vi "Exercise 4.3.vi"() -> ()   [LabVIEW 2010]
panel:
  in  "stop":bool
  in  "Left/Right":i32=-22
  in  "Up/Down":i32=-142
  in  "Scale 2":u32=29 min=1
  out "Intensity Graph":dbl[][](graph)
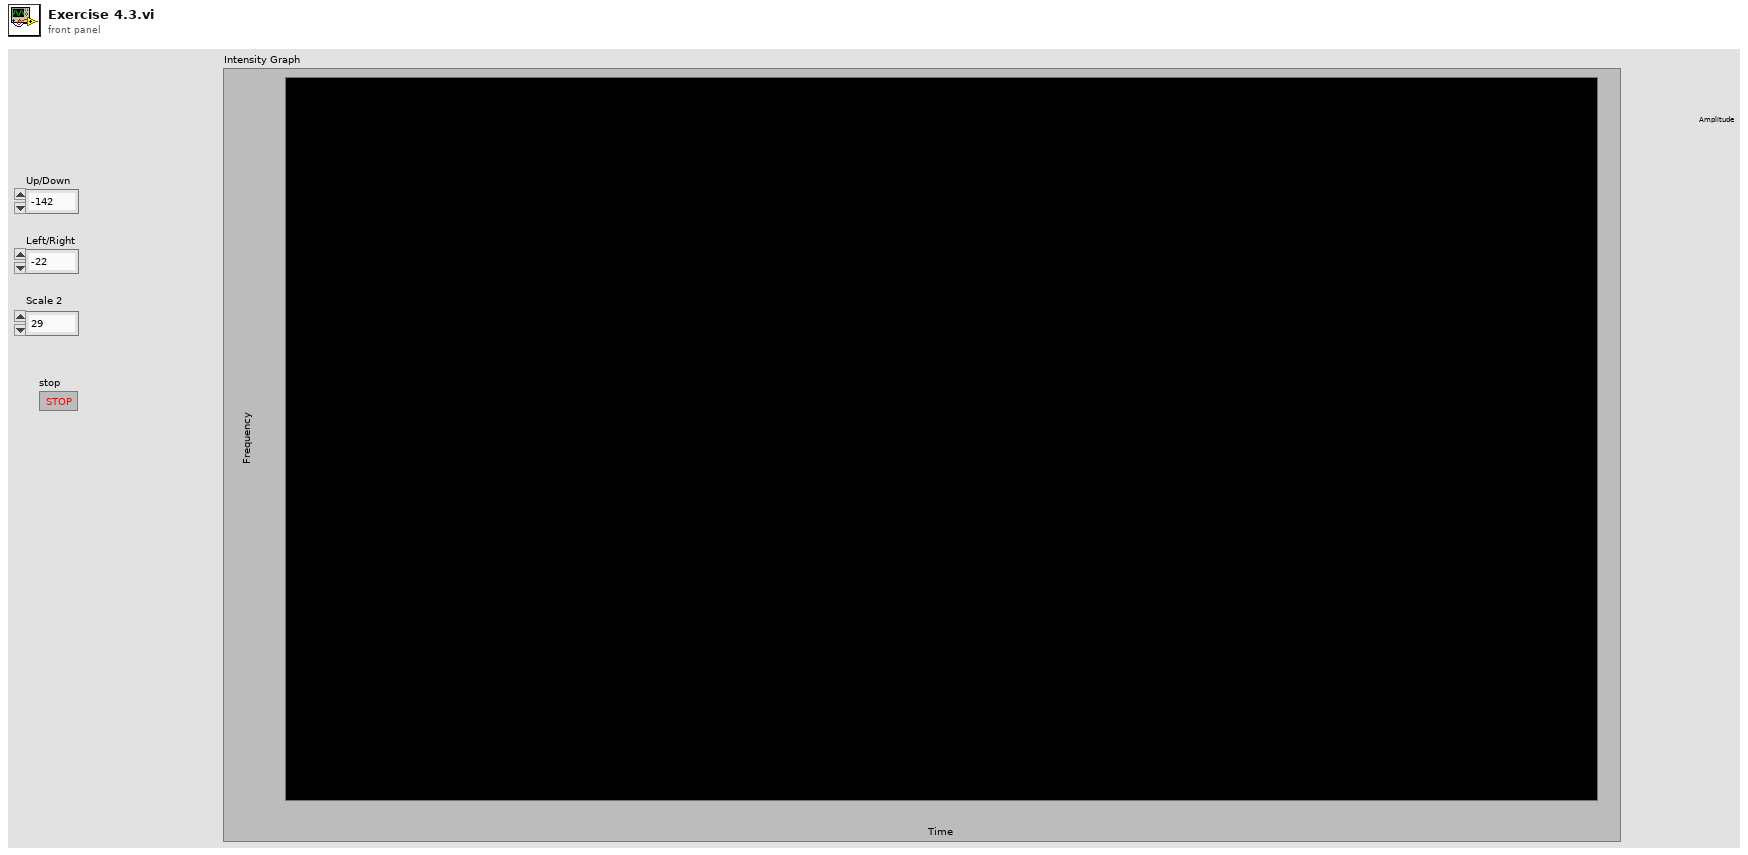
[diagram p1: front panel]
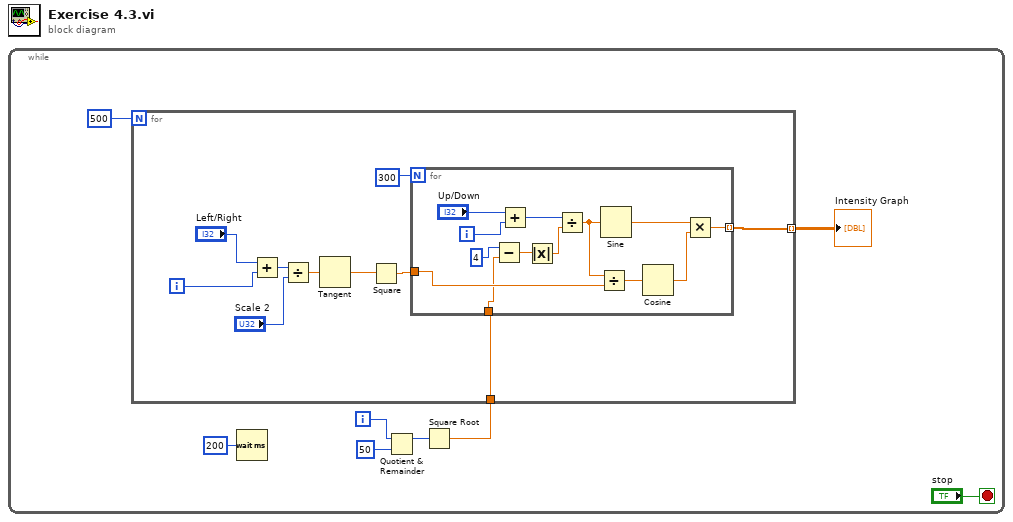
[diagram p0: block diagram]
diagram:
  n1 = while {
    i -> [w5]
    stop <- "stop" stop-if-true
    n2 = Wait (ms)(milliseconds to wait=u32 200) -> ()  [unwired: 1 out]
    n3 = Quotient & Remainder(x=w5, y=50) -> (x-y*floor(x/y)=w2:i32)  [unwired: 1 out]
    n4 = Square Root(x=w2) -> (sqrt(x)=w1:dbl)
    n5 = for {
      N: 500 -> [_]
      tunnel: [w17] -> w8 mode=indexing
      tunnel: w1 -> [w9]
      i -> [w10]
      n6 = Add(x="Left/Right", y=w10) -> (x+y=w11:i32)
      n7 = Divide(x=w11, y="Scale 2") -> (x/y=w15:dbl)
      n8 = Tangent(1:w15) -> (0:w14:dbl)
      n9 = Square(x=w14) -> (x^2=w13:dbl)
      n10 = for {
        N: 300 -> [_]
        tunnel: w13 -> [w29]
        tunnel: [w27] -> w17 mode=indexing
        tunnel: w9 -> [w19]
        i -> [w25]
        n11 = Subtract(x=4 ("y"), y=w19) -> (x-y=w22:dbl)
        n12 = Add(x="Up/Down", y=w25) -> (x+y=w23:i32)
        n13 = Absolute Value(x=w22) -> (abs(x)=w21:dbl)
        n14 = Divide(x=w23, y=w21) -> (x/y=w26:dbl)
        n15 = Divide(x=w26, y=w29) -> (x/y=w28:dbl)
        n16 = Sine(x=w26) -> (sin(x)=w31:dbl)
        n17 = Cosine(x=w28) -> (cos(x)=w30:dbl)
        n18 = Multiply(x=w31, y=w30) -> (x*y=w27:dbl)
      }
    }
    "Intensity Graph" <- w8
  }
